vi "CHD_TRAJECTORY_EXECUTE_REL.vi"(6 "Pass_Through_Time":dbl=-1.0 format="%33.4f", 8 "Init":bool, 11 "TrajectoryName":string) -> (1 "Complete":bool, 2 "AtReference":bool, 3 "Chassis Velocity Target SI":T1 {"vOmega" format="%10.3f"; "vY" format="%10.3f"; "vX" format="%10.3f"})   [LabVIEW 2019]
uses:
  CHD_TRAJECTORY_GLOBALS.vi
  <vilib>/Rock Robotics/WPI/ThirdParty/JAS_Junk/TrajLib/Trajectory_Library.lvlib
  <vilib>/Rock Robotics/WPI/ThirdParty/ChoreoLib/ChoreoLib.lvlib
  <vilib>/Rock Robotics/WPI/ThirdParty/JAS_Junk/TrajLib/TypeDef/CHASSIS_SPEEDS.ctl
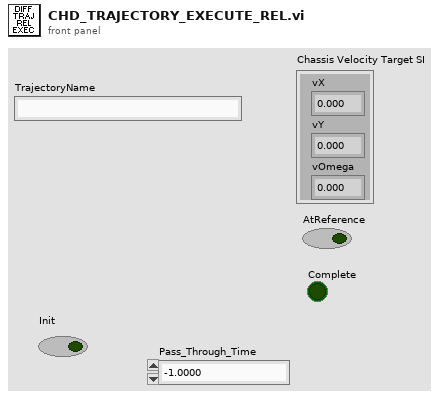
[diagram p1: front panel]
types:
  T1 = typedef "Trajectory_Library.lvlib/CHASSIS_SPEEDS.ctl" = cluster{"vX":dbl, "vY":dbl, "vOmega":dbl}
  T2 = typedef "Trajectory_Library.lvlib/ROTATION2D.ctl" = cluster{"VALUE":dbl, "COS":dbl, "SIN":dbl}
  T3 = typedef "Trajectory_Library.lvlib/POSE2D.ctl" = cluster{"TRANSLATION":T4, "ROTATION":T2}
  T4 = typedef "Trajectory_Library.lvlib/TRANSLATION2D.ctl" = cluster{"X":dbl, "Y":dbl}
  T5 = cluster{"X Pos Err M":dbl, "Y Pos Err M":dbl, "Rot Pos Err Deg":dbl}
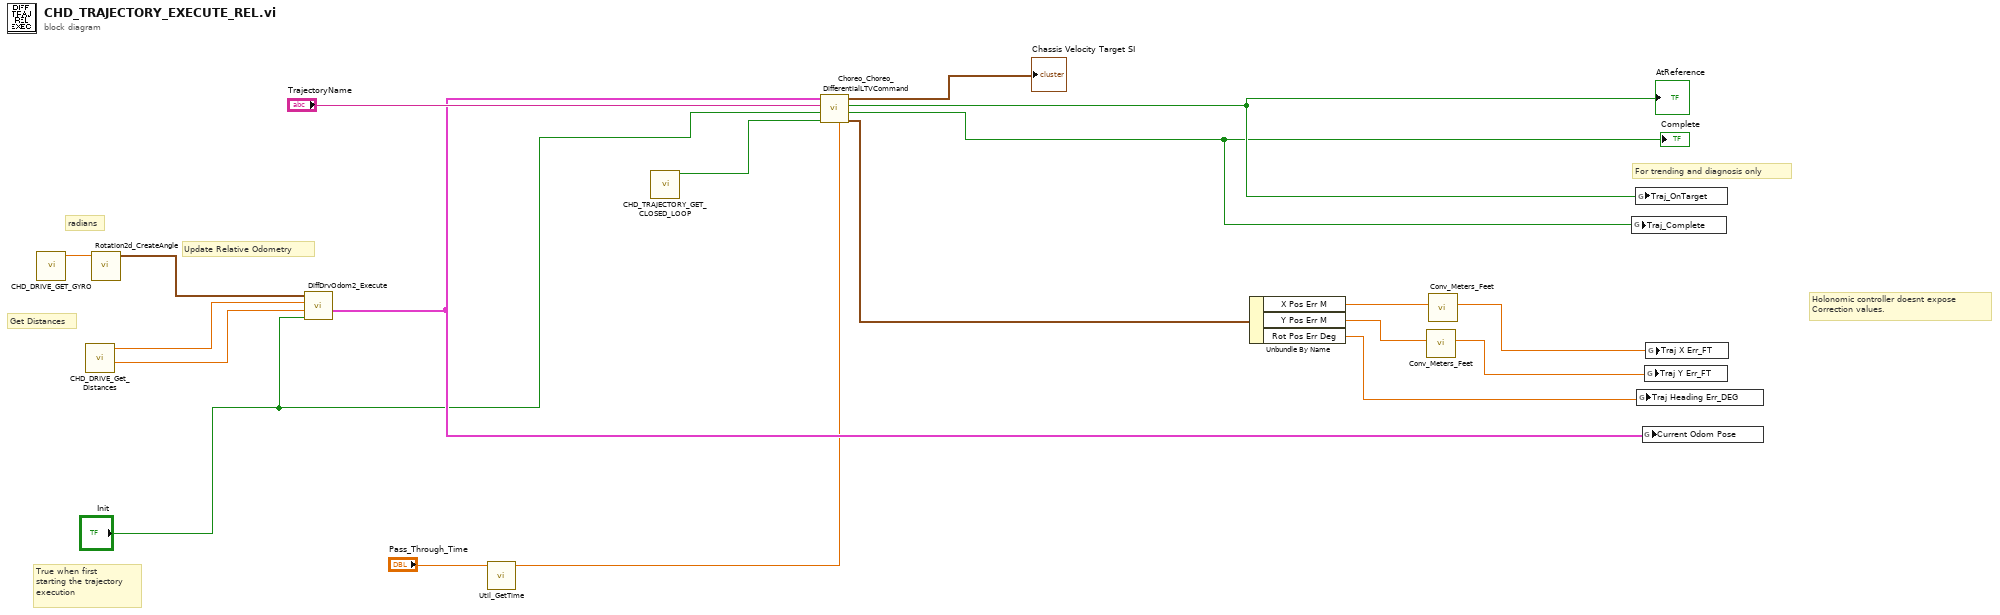
[diagram p0: block diagram]
diagram:
  # "Get Distances"
  # "Update Relative Odometry"
  # "radians"
  # "True when first\nstarting the trajectory\nexecution"
  # "Holonomic controller doesnt expose\nCorrection values."
  # "For trending and diagnosis only"
  n1 = call "CHD_DRIVE_GET_GYRO.vi"() -> ("Gyro Heading Radians"=w18:dbl)  [unwired: 11 in]
  n2 = call "CHD_DRIVE_Get_Distances.vi"() -> ("RightDistance_M"=w8:dbl, "LeftDistance_M"=w9:dbl)  [unwired: 9 in, 1 out]
  n3 = call <vilib>:"Rotation2d_CreateAngle.vi"("Angle"=w18) -> ("ROTATION"=w11:T2)  [unwired: 10 in]
  n4 = call <vilib>:"DiffDrvOdom2_Execute.vi"("Init / Reset"="Init", "Right Distance M"=w8, "Left Distance M"=w9, "Gyro Reading"=w11) -> ("Pose Meters"=w10:T3)  [unwired: 6 in, 1 out]
  n5 = call <vilib>:"Util_GetTime.vi"("Pass_Through_Time"="Pass_Through_Time") -> ("FPGA_Time_Seconds"=w1:dbl)  [unwired: 8 in, 2 out]
  n6 = call "CHD_TRAJECTORY_GET_CLOSED_LOOP.vi"() -> ("AUTO_CLOSED_LOOP"=w6:bool)  [unwired: 11 in]
  n7 = call <vilib>:"Choreo_Choreo_DifferentialLTVCommand.vi"("Pass_Through_Time"=w1, "Auto"=w6, "Initialize"="Init", "TrajectoryName"="TrajectoryName", "Current Position"=w10) -> ("Ctrl Info"=w2:T5, "Complete"=w3:bool, "On Target"=w4:bool, "Chassis Speed Dmd"=→"Chassis Velocity Target SI":T1)  [unwired: 3 in]
  "AtReference" <- w4
  "Complete" <- w3
  n8 = Unbundle By Name(w2) -> ("X Pos Err M"=w17:dbl, "Y Pos Err M"=w16:dbl, "Rot Pos Err Deg"=w13:dbl)
  n9 = call <vilib>:"Conv_Meters_Feet.vi"("Meters"=w16) -> ("Feet"=w14:dbl)  [unwired: 10 in]
  n10 = call <vilib>:"Conv_Meters_Feet.vi"("Meters"=w17) -> ("Feet"=w15:dbl)  [unwired: 10 in]
  n11 = global write "CHD_TRAJECTORY_GLOBALS.vi" "Traj_Complete"(w3) -> ()
  n12 = global write "CHD_TRAJECTORY_GLOBALS.vi" "Traj_OnTarget"(w4) -> ()
  n13 = global write "CHD_TRAJECTORY_GLOBALS.vi" "Traj Heading Err_DEG"(w13) -> ()
  n14 = global write "CHD_TRAJECTORY_GLOBALS.vi" "Current Odom Pose"(w10) -> ()
  n15 = global write "CHD_TRAJECTORY_GLOBALS.vi" "Traj Y Err_FT"(w14) -> ()
  n16 = global write "CHD_TRAJECTORY_GLOBALS.vi" "Traj X Err_FT"(w15) -> ()
